vi "Read Communications Configuration.vi"(8 "error in (no error)":errorcluster, 11 "Communications in":refnum<class "Communications.lvclass">) -> (0 "error out":errorcluster, 2 "Configuration":T1={"Subscribe to modules"=["Spectrum Recorder", "Line Detector"]}, 3 "Communications out":refnum<class "Communications.lvclass">)   [LabVIEW 2019, in "Communications.lvclass"]
uses:
  Communications.lvclass
  Communications Configuration.ctl
  Communications.lvclass/Communications.ctl
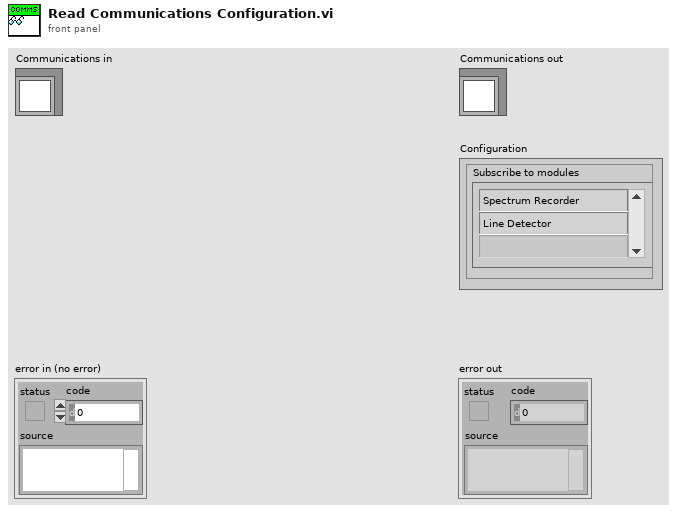
[diagram p1: front panel]
types:
  T1 = typedef "Communications Configuration.ctl" = cluster{"Subscribe to modules":string[]}
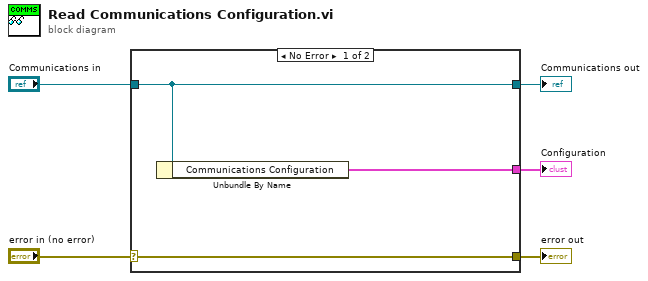
[diagram p0: block diagram]
diagram:
  n1 = case shown="No Error" "error in (no error)" {
    selector: "error in (no error)" -> [w8 w9]
    tunnel: [w8 w9] -> w4
    tunnel: [w7 w10] -> w2
    tunnel: "Communications in" -> [w7 w10]
    tunnel: [w6 _] -> w1
    frame No Error {
      n2 = Unbundle By Name(w7) -> ("Communications Configuration"=w6:T1)
    }
    frame Error {
    }
  }
  "error out" <- w4
  "Communications out" <- w2
  "Configuration" <- w1
